vi "Get DSP Version.vi"(5 "Delay Time (s)":dbl) -> (0 "error out":errorcluster, 1 "return value":i32, 2 "DSP version":string)   [LabVIEW 2015]
uses:
  ScannerDiagDLL.dll
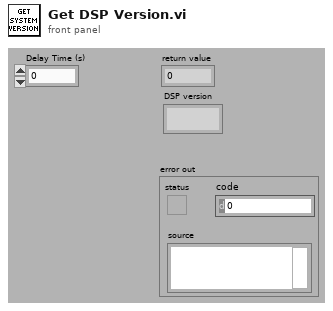
[diagram p1: front panel]
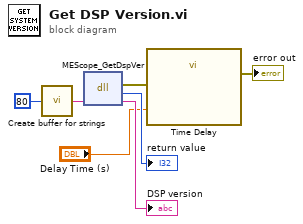
[diagram p0: block diagram]
diagram:
  n1 = call "Create buffer for strings.vi"("# of spaces"=80) -> ("String Buffer"=w6:string)  [unwired: 4 in]
  n2 = dll-call lib="C:/SNAPON/ModisEdge/TabletScope/Test Sequence/Code Modules/DLL/ScannerDiagDLL.dll" fn="MEScope_GetDspVer"("szTargBuff"=w6) -> (error out=w4:errorcluster, "return type"=→"return value":i32, "szTargBuff"=→"DSP version":string)  [unwired: 3 in, 1 out]
  n3 = call "Time Delay"("error in (no error)"=w4, "Delay Time (s)"="Delay Time (s)") -> ("error out"=→"error out":errorcluster)  [unwired: 9 in]
